vi "Check Data Model.vi"(8 "error in (no error)":errorcluster, 11 "device data model in":refnum<class "ICPCON PM3114 Data Model.lvclass">) -> (0 "error out":errorcluster, 3 "device data model out":refnum<class "ICPCON PM3114 Data Model.lvclass">)   [LabVIEW 2021, in "ICPCON PM3114 Data Model.lvclass"]
doc: "This VI ensures that the data model has at least 65,535 values of every type. This is required for certain modbus function codes."
uses:
  ICPCON PM3114 Data Model.lvclass
  ICPCON PM3114 Data Model.lvclass/ICPCON PM3114 Data Model.ctl
  Type Definitions/Data Model.ctl
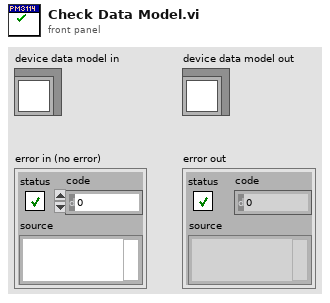
[diagram p1: front panel]
types:
  T1 = typedef "ICPCON PM3114 Data Model.lvclass/Data Model.ctl" = cluster{"UTC":u64, "Power value":sgl[], "ES":u8}
  T2 = typedef "Device Data Model.lvclass/N channel.ctl" = cluster{"N DI channel":i32, "N DO channel":i32, "N AI channel":i32, "N AO channel":i32}
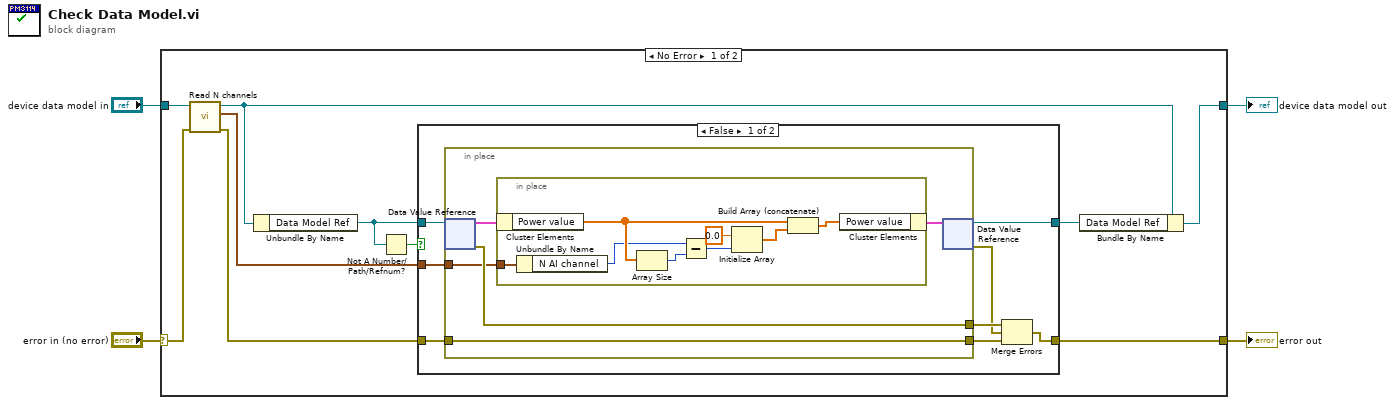
[diagram p0: block diagram]
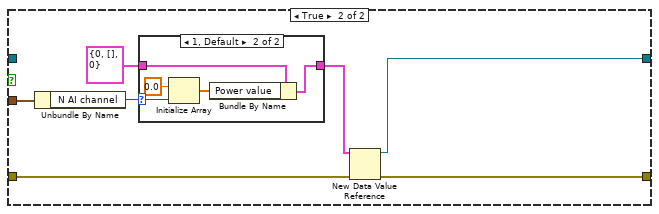
[diagram p2: hidden frame]
diagram:
  n1 = case shown="No Error" "error in (no error)" {
    selector: "error in (no error)" -> [w7 w50]
    tunnel: "device data model in" -> [w9 w49]
    tunnel: [w14 w49] -> w3
    tunnel: [w10 w50] -> w2
    frame No Error {
      n2 = call-dynamic "Read N channels.vi"("error in (no error)"=w7, "device data model in"=w9) -> ("error out"=w6:errorcluster, "N channel"=w5:T2, "device data model out"=w8:refnum<class "ICPCON PM3114 Data Model.lvclass">)  [unwired: 7 in]
      n3 = Unbundle By Name(w8) -> ("Data Model Ref"=w12:refnum<data-value>)
      n4 = Not A Number/Path/Refnum?(number/path/refnum=w12) -> (NaN/Path/Refnum?=w11:bool)
      n5 = case shown="False" w11 {
        tunnel: w6 -> [w22 w42]
        tunnel: w12 -> [w21 _]
        tunnel: [w20 w40] -> w13
        tunnel: [w18 w41] -> w10
        tunnel: w5 -> [w15 w37]
        frame False {
          n6 = in-place {
            in-place-border: w22 -> [w25]
            in-place-border: [w26] -> w19
            in-place-border: [w25] -> w16
            in-place-border: w15 -> [w24]
            n7 = in-place-dvr #1(w21) -> (w27:T1, w26:errorcluster)
            n8 = in-place {
              in-place-border: w24 -> [w29]
              n9 = in-place-cluster #2(w27) -> ("Power value"=w32:sgl[])
              n10 = Unbundle By Name(w29) -> ("N AI channel"=w28:i32)
              n11 = Array Size(array=w32) -> (size(s)=w35:i32)
              n12 = Subtract(x=w28, y=w35) -> (x-y=w34:i32)
              n13 = Initialize Array(sgl 0.0 ("Boolean"), w34) -> (w33:sgl[])
              n14 = Build Array (concatenate)(w32, w33) -> (w30:sgl[])
              n15 = in-place-cluster #2("Power value"=w30) -> (w23:T1)
            }
            n16 = in-place-dvr #1(w23) -> (w20:refnum<data-value>, w17:errorcluster)
          }
          n17 = Merge Errors(w19, w17, w16) -> (w18:errorcluster)
        }
        frame True {
          n18 = Unbundle By Name(w37) -> ("N AI channel"=w38:i32)
          n19 = case shown="1, Default" w38 {
            selector: w38 -> [_ w44]
            tunnel: T1 {"UTC"=0, "Power value"=[], "ES"=0} ("Data Model") -> [w43 w47]
            tunnel: [w43 w45] -> w36
            frame 0 {
            }
            frame 1, Default {
              n20 = Initialize Array(sgl 0.0 ("Boolean"), w44) -> (w46:sgl[])
              n21 = Bundle By Name(cluster=w47, "Power value"=w46) -> (w45:T1)
            }
          }
          n22 = New Data Value Reference(data value=w36, error in=w42) -> (data value reference=w40:refnum<data-value>, error out=w41:errorcluster)
        }
      }
      n23 = Bundle By Name(cluster=w8, "Data Model Ref"=w13) -> (w14:refnum<class "ICPCON PM3114 Data Model.lvclass">)
    }
    frame Error {
    }
  }
  "error out" <- w2
  "device data model out" <- w3
